vi "New RegWrite Command.vi"(0 "RFFE RegWrite Command in":refnum<class "RFFE RegWrite Command.lvclass">, 5 "Slave Address":T3=12 format="%02x", 7 "Register Address":T2 format="%02x", 9 "Register Data":T1 format="%02x", 11 "error in (no error)":errorcluster) -> (4 "RFFE RegWrite Command out":refnum<class "RFFE RegWrite Command.lvclass">, 15 "error out":errorcluster)   [LabVIEW 2018, in "MIPI RFFE API.lvlib" / "RFFE RegWrite Command.lvclass"]
uses:
  RFFE RegWrite Command.lvclass
  C:/Users/semoore/Projects/mipi-rffe-labview-oop/Standard Command/RFFE Standard Command.lvclass
  Slave Address.ctl
  Register Address.ctl
  Register Data.ctl
  Standard Command/RFFE Standard Command.lvclass
  MIPI RFFE API.lvlib
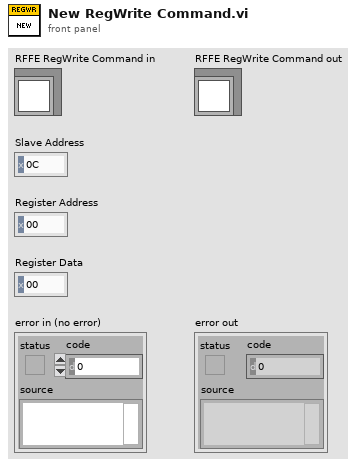
[diagram p1: front panel]
types:
  T1 = typedef "MIPI RFFE API.lvlib/Register Data.ctl" = u8
  T2 = typedef "MIPI RFFE API.lvlib/Register Address.ctl" = u16
  T3 = typedef "MIPI RFFE API.lvlib/Slave Address.ctl" = u8
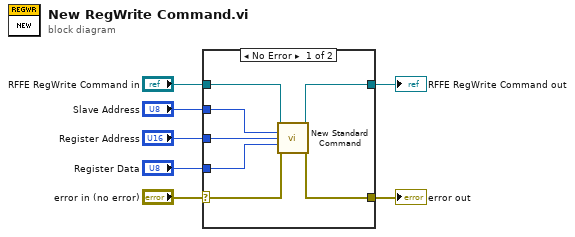
[diagram p0: block diagram]
diagram:
  n1 = case shown="No Error" "error in (no error)" {
    selector: "error in (no error)" -> [w12 w16]
    tunnel: [w11 w16] -> w6
    tunnel: [w14 w15] -> w4
    tunnel: "RFFE RegWrite Command in" -> [w13 w15]
    tunnel: "Register Data" -> [w10 _]
    tunnel: "Register Address" -> [w9 _]
    tunnel: "Slave Address" -> [w8 _]
    frame No Error {
      n2 = call "New Standard Command.vi"("RFFE Standard Command in"=w13, "Slave Address"=w8, "Register Address"=w9, "Register Data"=w10, "error in (no error)"=w12) -> ("RFFE Standard Command out"=w14:refnum<class "RFFE RegWrite Command.lvclass">, "error out"=w11:errorcluster)  [unwired: 9 in]
    }
    frame Error {
    }
  }
  "error out" <- w6
  "RFFE RegWrite Command out" <- w4
